vi "Value Strings.vi"(8 "error in (no error)":errorcluster, 11 "StringGroup in":refnum<class "Group STR.lvclass">) -> (0 "error out":errorcluster, 1 "Timestamps":dbl[](array[numeric]), 2 "Value Strings":string[](array[string]), 3 "StringGroup out":refnum<class "Group STR.lvclass">)   [LabVIEW 2020, in "Vecto.lvlib" / "Group STR.lvclass"]
uses:
  Group STR.lvclass
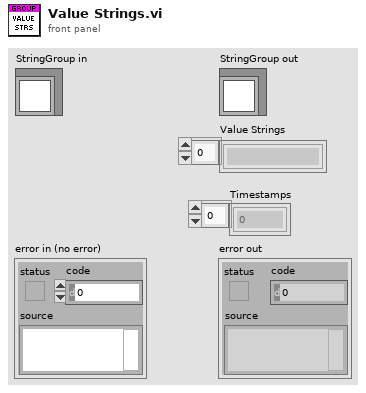
[diagram p1: front panel]
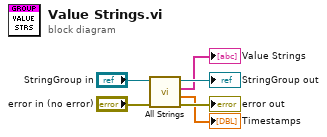
[diagram p0: block diagram]
diagram:
  n1 = call "All Strings.vi"("error in (no error)"="error in (no error)", "StringGroup in"="StringGroup in") -> ("error out"=→"error out":errorcluster, "Timestamps"=→"Timestamps":dbl[], "Strings"=→"Value Strings":string[], "StringGroup out"=→"StringGroup out":refnum<class "Group STR.lvclass">)  [unwired: 6 in]
